vi "Begin.vi"() -> (0 "error out":errorcluster)   [LabVIEW 2013]
doc: "Called before other user functions, this VI is expected to open initial I/O refnums, load in file data, and do all program initialization. Notice that the <B>error out</B> terminal is simply used for data flow. Wiring it to other structures or subVIs ensures that this VI runs first."
uses:
  <vilib>/Rock Robotics/WPI/DriverStation/WPI_DriverStationRobotMode2.ctl
  Physical Systems/XBoxController/XBoxController-P.lvclass
  <vilib>/ActorFramework/Message Queue/Message Queue.lvclass/Message Queue.ctl
  Robot Global Data.vi
  <vilib>/ActorFramework/Actor/Actor.lvclass
  <vilib>/ActorFramework/Message Queue/Message Queue.lvclass
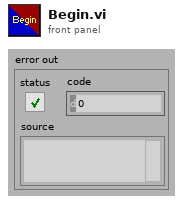
[diagram p1: front panel]
types:
  T1 = typedef "WPI_DriverStationRobotMode2.ctl" = enum16{"Autonomous Disabled", "Autonomous Enabled", "Teleop Disabled", "Teleop Enabled", "Timeout", "Finish", "Test Disabled", "Test Enabled"}
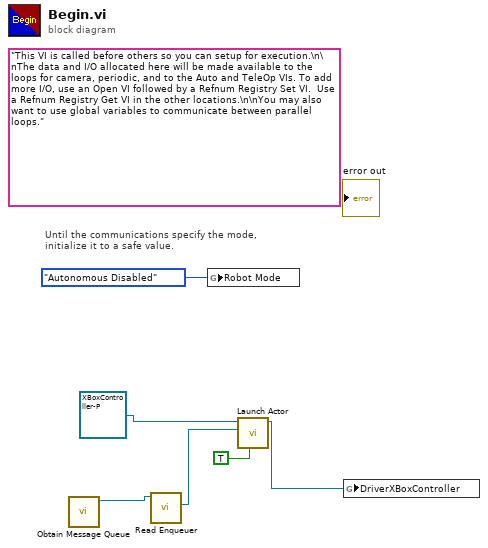
[diagram p0: block diagram]
diagram:
  (unwired) "This VI is called before others so you can setup for execution.\n\nThe data and I/O allocated here will be made available to the loops for camera, periodic, and to the Auto and TeleOp VIs. To add more I/O, use an Open VI followed by a Refnum Registry Set VI.  Use a Refnum Registry Get VI in the other locations.\n\nYou may also want to use global variables to communicate between parallel loops."
  # "Until the communications specify the mode,\ninitialize it to a safe value."
  n1 = call <vilib>:"Obtain Message Queue.vi"() -> ("Message Queue"=w5:refnum<class "Message Queue.lvclass">)  [unwired: 10 in, 1 out]
  n2 = call <vilib>:"Read Enqueuer.vi"("Message Queue"=w5) -> ("Message Enqueuer"=w4:refnum<class "Message Enqueuer.lvclass">)  [unwired: 10 in]
  n3 = global write "Robot Global Data.vi" "Robot Mode"(WPI_DriverStationRobotMode2."Autonomous Disabled" ("Robot Mode")) -> ()
  n4 = call <vilib>:"Launch Actor.vi"("Open Actor Core front panel? (F)"=TRUE, "Actor-to-Caller Enqueuer"=w4, "Actor"=refnum<class "XBoxController-P.lvclass"> refnum ("XBoxController-P.lvclass")) -> ("Caller-To-Actor Enqueuer"=w2:refnum<class "Message Enqueuer.lvclass">)  [unwired: 7 in, 1 out]
  n5 = global write "Robot Global Data.vi" "DriverXBoxController"(w2) -> ()
